vi "下降沿 (子VI).vi"(10 "Last Signal":bool, 11 "Signal":bool) -> (3 "Down?":bool)   [LabVIEW 2017]
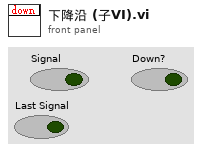
[diagram p1: front panel]
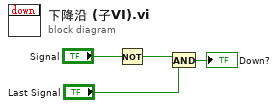
[diagram p0: block diagram]
diagram:
  n1 = Not(x="Signal") -> (.not. x?=w2:bool)
  n2 = And(x=w2, y="Last Signal") -> (x .and. y?=→"Down?":bool)
